vi "deleteState History.vi"(5 "Current State in":string) -> (2 "State History":string)   [LabVIEW 2019]
uses:
  Instrument.Lockin.lvclass
panel:
  out "Current State out":string
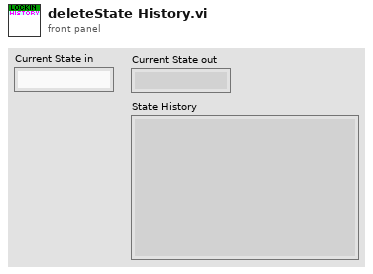
[diagram p1: front panel]
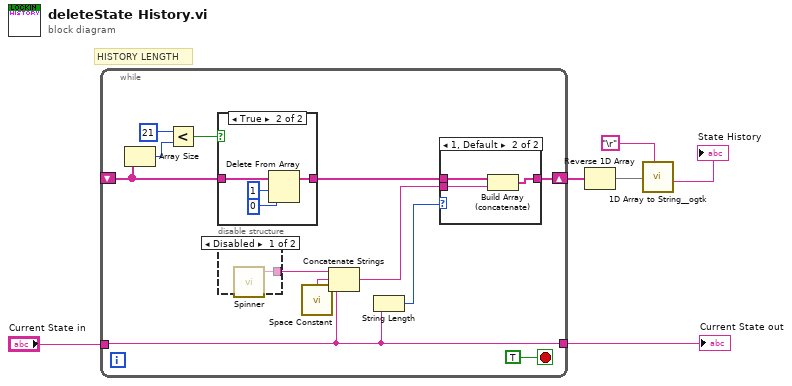
[diagram p0: block diagram]
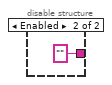
[diagram p2: hidden frame]
diagram:
  # "HISTORY LENGTH"
  n1 = while {
    tunnel: "Current State in" -> [w12]
    tunnel: [w12] -> w6
    shift-right: [w13] -> w2
    shift-left: _ -> [w14]
    stop <- TRUE stop-if-true
    n2 = Array Size(array=w14) -> (size(s)=w17:i32)
    n3 = Less?(x=21 ("length"), y=w17) -> (x < y?=w9:bool)
    n4 = case shown="True" w9 {
      tunnel: w14 -> [w25 w26]
      tunnel: [w25 w28] -> w18
      frame False {
      }
      frame True {
        n5 = Delete From Array(array=w26, length=1, index=0) -> (array with subset deleted=w28:string[])  [unwired: 1 out]
      }
    }
    n6 = disable-structure shown="Disabled" {
      disable-tunnel: [w19 "" ("Spinner Out")] -> w11
      frame Disabled {
        n7 = call "Spinner.vi"() -> ("Spinner Out"=w19:string)  [unwired: 5 in]
      }
      frame Enabled {
      }
    }
    n8 = call <vilib>:"Space Constant.vi"() -> ("String"=w10:string)
    n9 = Concatenate Strings(w11, w10, w12) -> (w8:string)
    n10 = String Length(string=w12) -> (length=w7:i32)
    n11 = case shown="1, Default" w7 {
      tunnel: w18 -> [w21 w23]
      tunnel: [w21 w24] -> w13
      tunnel: w8 -> [_ w22]
      frame 0 {
      }
      frame 1, Default {
        n12 = Build Array (concatenate)(w23, w22) -> (w24:string[])
      }
    }
  }
  "Current State out" <- w6
  n13 = Reverse 1D Array(array=w2) -> (reversed array=w1:string[])
  n14 = call <userlib>:"1D Array to String__ogtk.vi"("delimiter (Tab)"="\r", "Array of Strings"=w1) -> ("delimited string"=→"State History":string)  [unwired: 9 in]
